vi "update_coag_dose.vi"(11 "Input Array":dbl[](array[numeric])) -> (2 "Coagulant_dose [mg/L]":dbl)   [LabVIEW 2019]
uses:
  RowData_Type.ctl
  Global Plantita Parameters.vi
  store_last_RowData.vi
panel:
  out "Added Row Display":T1
  out "Data buffer length":dbl
  out "Display":T1[](array[typedef])
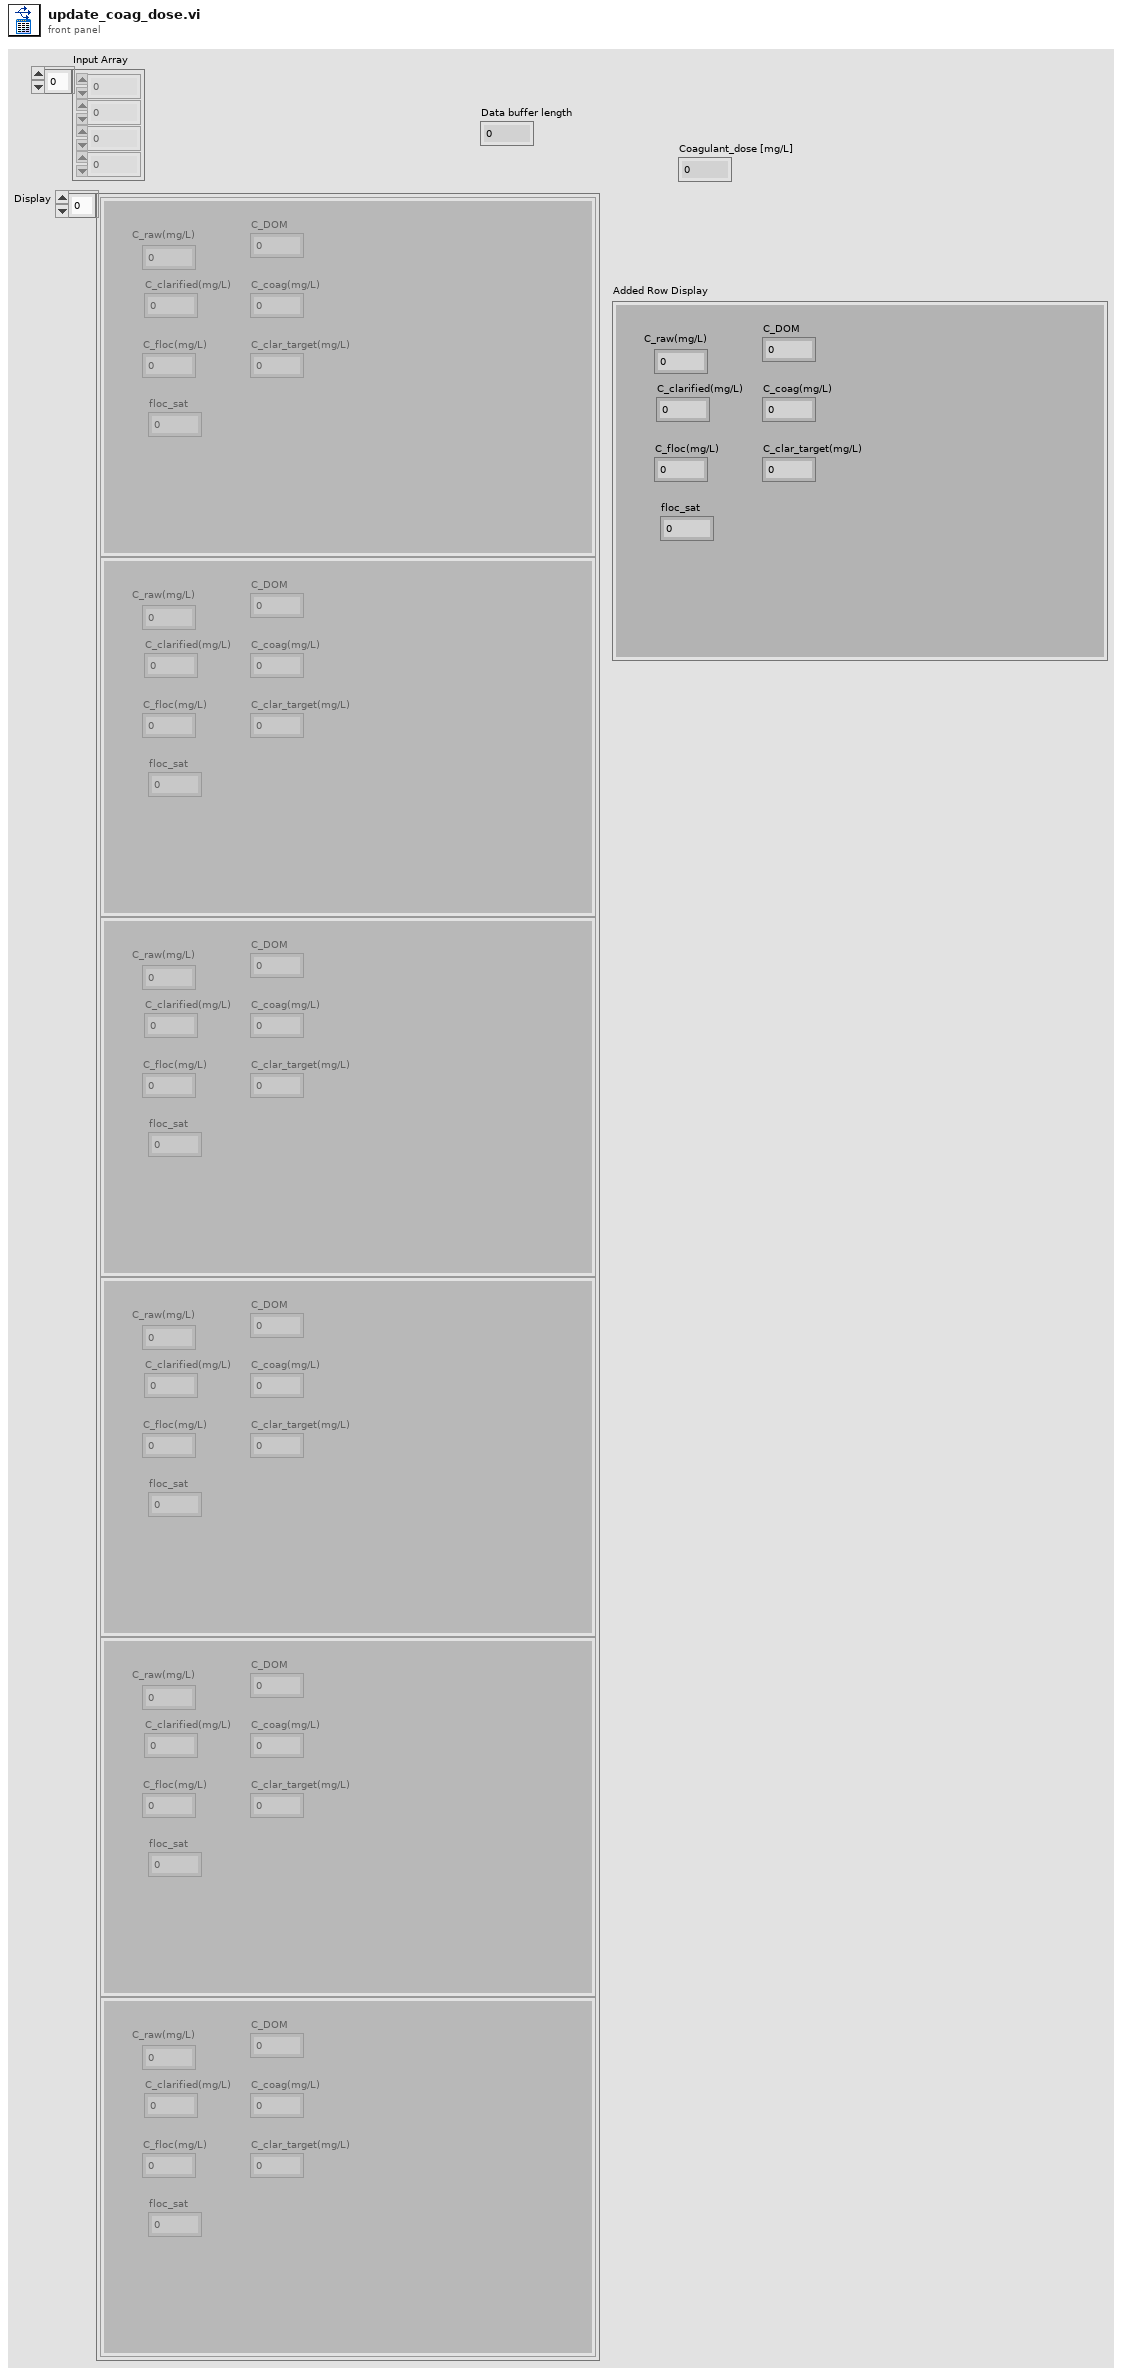
[diagram p1: front panel]
types:
  T1 = typedef "RowData_Type.ctl" = cluster{"C_raw(mg/L)":dbl, "C_clarified(mg/L)":dbl, "C_floc(mg/L)":dbl, "floc_sat":dbl, "C_DOM":dbl, "C_coag(mg/L)":dbl, "C_clar_target(mg/L)":dbl}
  T2 = cluster{"height_ff (m)":dbl, "C_coag_stock (g/L)":dbl, "flocculation_time(min)":dbl, "clarification_time(min)":dbl, "data_interval (min)":dbl, "kpf":dbl, "kc":dbl, "q":dbl}
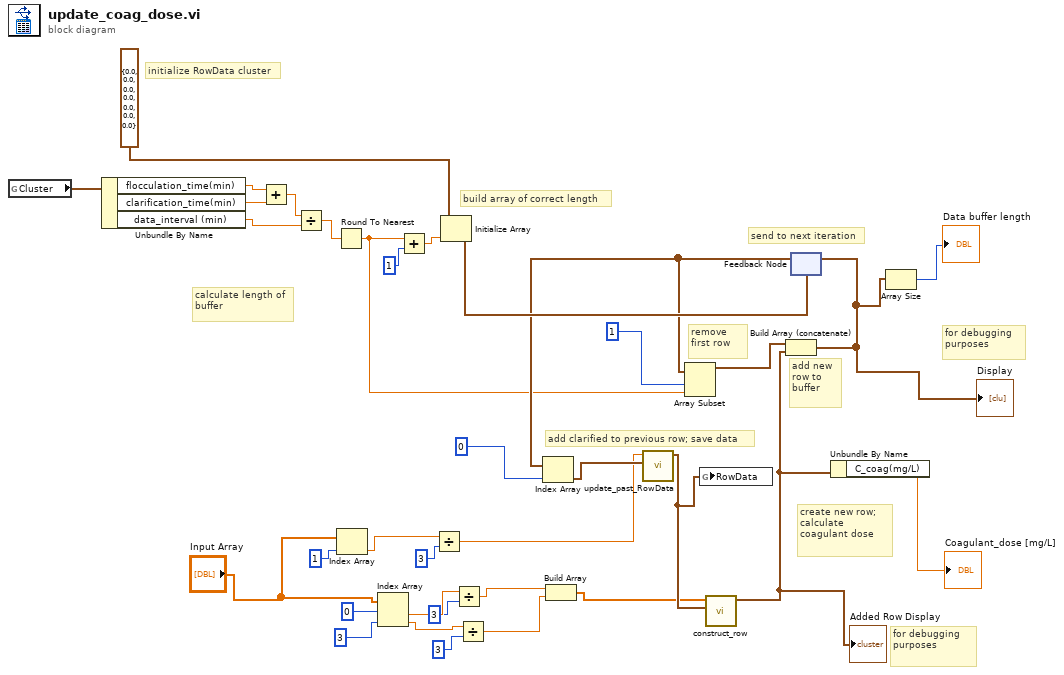
[diagram p0: block diagram]
diagram:
  # "for debugging purposes"
  # "remove first row"
  # "add new row to buffer"
  # "create new row;\ncalculate coagulant dose"
  # "add clarified to previous row; save data"
  # "send to next iteration"
  # "build array of correct length"
  # "initialize RowData cluster"
  # "calculate length of buffer"
  # "for debugging purposes"
  n1 = global read "Global Plantita Parameters.vi" "Cluster"() -> (w25:T2)
  n2 = Unbundle By Name(w25) -> ("flocculation_time(min)"=w24:dbl, "clarification_time(min)"=w23:dbl, "data_interval (min)"=w21:dbl)
  n3 = Add(x=w24, y=w23) -> (x+y=w22:dbl)
  n4 = Divide(x=w22, y=w21) -> (x/y=w20:dbl)
  n5 = Round To Nearest(number=w20) -> (nearest integer value=w2:dbl)
  n6 = Index Array(array="Input Array", index=1) -> (element=w16:dbl)
  n7 = Index Array(array="Input Array", index #1=0, index #2=3) -> (element #1=w10:dbl, element #2=w7:dbl)
  n8 = Add(x=w2, y=1) -> (x+y=w1:dbl)
  n9 = Divide(x=w16, y=3) -> (x/y=w14:dbl)
  n10 = Initialize Array(T1 {"C_raw(mg/L)"=0.0, "C_clarified(mg/L)"=0.0, "C_floc(mg/L)"=0.0, "floc_sat"=0.0, "C_DOM"=0.0, "C_coag(mg/L)"=0.0, "C_clar_target(mg/L)"=0.0} ("typedef_test"), w1) -> (w35:T1[])
  n11 = Divide(x=w10, y=3) -> (x/y=w6:dbl)
  n12 = Divide(x=w7, y=3) -> (x/y=w5:dbl)
  n13 = Build Array(w6, w5) -> (w4:dbl[])
  n14 = feedback #1(w35) -> (w30:T1[])
  n15 = Index Array(array=w30, index=0) -> (element=w29:T1)
  n16 = call "update_past_RowData.vi"("RowData input"=w29, "Clarified turbidity (mg/L)"=w14) -> ("RowData output"=w26:T1)  [unwired: 9 in]
  n17 = Array Subset(array=w30, index=1, length=w2) -> (w33:T1[])
  n18 = global write "store_last_RowData.vi" "RowData"(w26) -> ()
  n19 = call "construct_row.vi"("input"=w26, "Array with C_raw, C_target"=w4) -> ("output"=w19:T1)  [unwired: 9 in]
  "Added Row Display" <- w19
  n20 = Build Array (concatenate)(w33, w19) -> (w18:T1[])
  "Display" <- w18
  n21 = feedback-in #1(w18) -> ()
  n22 = Unbundle By Name(w19) -> ("C_coag(mg/L)"=→"Coagulant_dose [mg/L]":dbl)
  n23 = Array Size(array=w18) -> (size(s)=→"Data buffer length":i32)
